vi "Set Default.vi"(8 "error in (no error)":errorcluster, 11 "Display Pop Up Msg in":refnum<class "Display Pop Up Msg.lvclass">) -> (0 "error out":errorcluster, 3 "Display Pop Up Msg out":refnum<class "Display Pop Up Msg.lvclass">)   [LabVIEW 2020, in "Msg.lvlib" / "Display Pop Up Msg.lvclass"]
doc: "Restore private data to a defined default state.\n\nThis implementation sets:\nPause time = -1\nPause? = TRUE"
uses:
  Display Pop Up Msg.lvclass
  Display Pop Up Msg.lvclass/Display Pop Up Msg.ctl
  Flex Msg/Flex Msg.lvclass
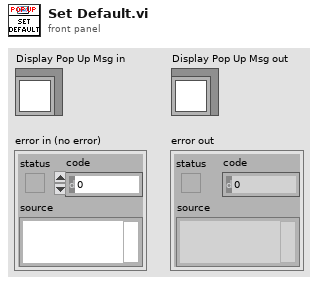
[diagram p1: front panel]
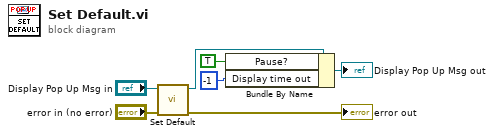
[diagram p0: block diagram]
diagram:
  n1 = call-parent "Set Default.vi"("error in (no error)"="error in (no error)", "Flex Msg in"="Display Pop Up Msg in") -> ("error out"=→"error out":errorcluster, "Flex Msg out"=w6:refnum<class "Display Pop Up Msg.lvclass">)  [unwired: 8 in]
  n2 = Bundle By Name(cluster=w6, "Pause?"=TRUE, "Display time out"=-1 ("Pause time out")) -> (→"Display Pop Up Msg out":refnum<class "Display Pop Up Msg.lvclass">)
